vi "Stop Core.vi"(10 "final error code":i32, 11 "output_poller in":refnum<class "output_poller.lvclass">) -> (3 "output_poller out":refnum<class "output_poller.lvclass">)   [LabVIEW 2015, in "output_poller.lvclass"]
doc: "(<B>Filename</B>: Actor Framework.lvlib:Actor.lvclass:Stop Core.vi)\n\nDefines what the actor does before it stops. Use the <B>final error code</B> input to determine whether the actor shut down in response to an error.\n\nBy default, this method does nothing. A descendant class may override it to define behavior, such as shutting down any processes the actor initiated in its override of the Actor Core method."
uses:
  output_poller.lvclass
  output_poller.lvclass/output_poller.ctl
  <vilib>/ActorFramework/Actor/Actor.lvclass
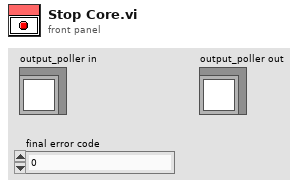
[diagram p1: front panel]
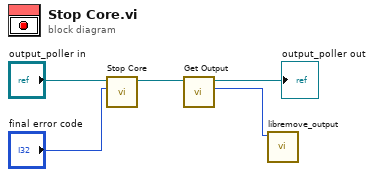
[diagram p0: block diagram]
diagram:
  n1 = call-parent "Stop Core.vi"("final error code"="final error code", "Actor in"="output_poller in") -> ("Actor out"=w3:refnum<class "output_poller.lvclass">)  [unwired: 9 in]
  n2 = call "Get Output.vi"("output_request_poller in"=w3) -> ("output"=w1:i32, "output_request_poller out"=→"output_poller out":refnum<class "output_poller.lvclass">)  [unwired: 8 in, 1 out]
  n3 = call "libremove_output.vi"("output"=w1) -> ()  [unwired: 10 in, 1 out]
